vi "Translate Into Error 5534.vi"(0 "error in (no error)":errorcluster, 1 "name":string) -> (2 "error out":errorcluster)   [LabVIEW 2015, in "Gates.lvlib"]
doc: "Translates from a queue-specific error into a gate-specific error if requested queue does not exists (original error code: 1100)."
uses:
  Gates.lvlib
  <vilib>/Utility/error.llb/Error Cluster From Error Code.vi
  <vilib>/ErrorRing/Error Ring.xnode
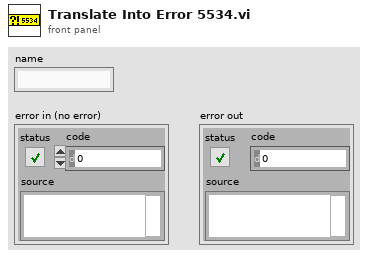
[diagram p1: front panel]
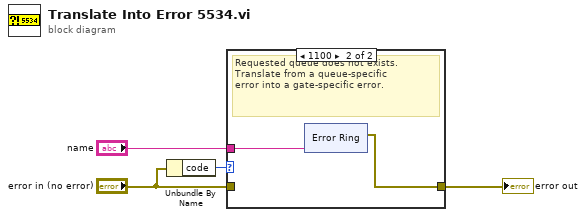
[diagram p0: block diagram]
diagram:
  n1 = Unbundle By Name("error in (no error)") -> ("code"=w1:i32)
  n2 = case shown="1100" w1 {
    tunnel: "name" -> [_ w7]
    tunnel: "error in (no error)" -> [w5 _]
    tunnel: [w5 w6] -> w4
    frame Default {
      # "Pass the error without modifications."
    }
    frame 1100 {
      # "Requested queue does not exists.\nTranslate from a queue-specific\nerror into a gate-specific error."
      n3 = xnode "Error Ring"("parameter 0"=w7) -> ("error out"=w6:errorcluster)
    }
  }
  "error out" <- w4
